vi "Init.vi"(11 "Game Play Type":refnum<vi>) -> (3 "cluster out":T1)   [LabVIEW 2019]
uses:
  Main VI references.ctl
  main queue data type.ctl
  top level commands.ctl
  error module commands.ctl
  Scene Commands.ctl
  Cube Data Ops.ctl
  Stop Timing Module commands.vi
  Play timing module commands.ctl
panel:
  in  "cluster":T1
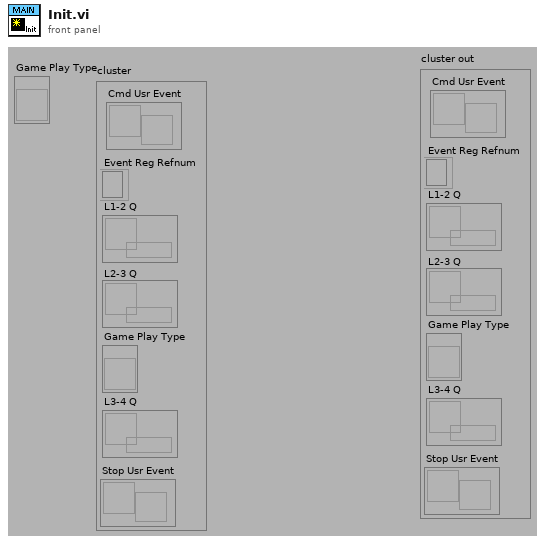
[diagram p1: front panel]
types:
  T1 = typedef "Main VI references.ctl" = cluster{"Cmd Usr Event":refnum<user-event>, "Event Reg Refnum":refnum<event-registration>, "L1-2 Q":refnum<queue>, "L2-3 Q":refnum<queue>, "Game Play Type":refnum<vi>, "L3-4 Q":refnum<queue>, "Stop Usr Event":refnum<user-event>}
  T2 = typedef "error module commands.ctl" = enum16{"Cleanup References", "Set References", "Report Errors", "Process Errors"}
  T3 = typedef "Scene Commands.ctl" = enum16{"Init", "Set Rubix Text Array", "Get Rubix Ref Array", "Generate Rubix Array", "Get Rubix Array", "Show Render Window", "Go To Face", "Rotate", "Update Scene", "Clear Rubix"}
  T4 = typedef "Play timing module commands.ctl" = enum16{"Clean up", "Initialize", "Run"}
  T5 = typedef "Cube Data Ops.ctl" = enum16{"Initialize", "Set Rubix Ref Array", "Set Rubix Text Array", "Set Current Face", "Get Rubix Text Array", "Generate Rubix Array", "Get Rubix array", "Get Facets to move", "Randomize", "Top row left", "Top row right", "Middle row left", "Middle row right", "Bottom row left", "Bottom row right", "Left column up", "Left column down", "Middle column up", "Middle column down", "Right column up", "Right column down", "Face ccw", "Face cw"}
  T6 = typedef "Stop Timing Module commands.vi" = enum16{"Set Name", "Stop loops"}
  T7 = typedef "main queue data type.ctl" = cluster{"Command":T8, "Data":variant}
  T8 = typedef "top level commands.ctl" = enum16{"Idle", "Set Cube Orientation", "Get Cube Orientation", "Go to Face", "Solve", "Test", "Randomize", "Game Play Type", "Stop", "rotate Cube"}
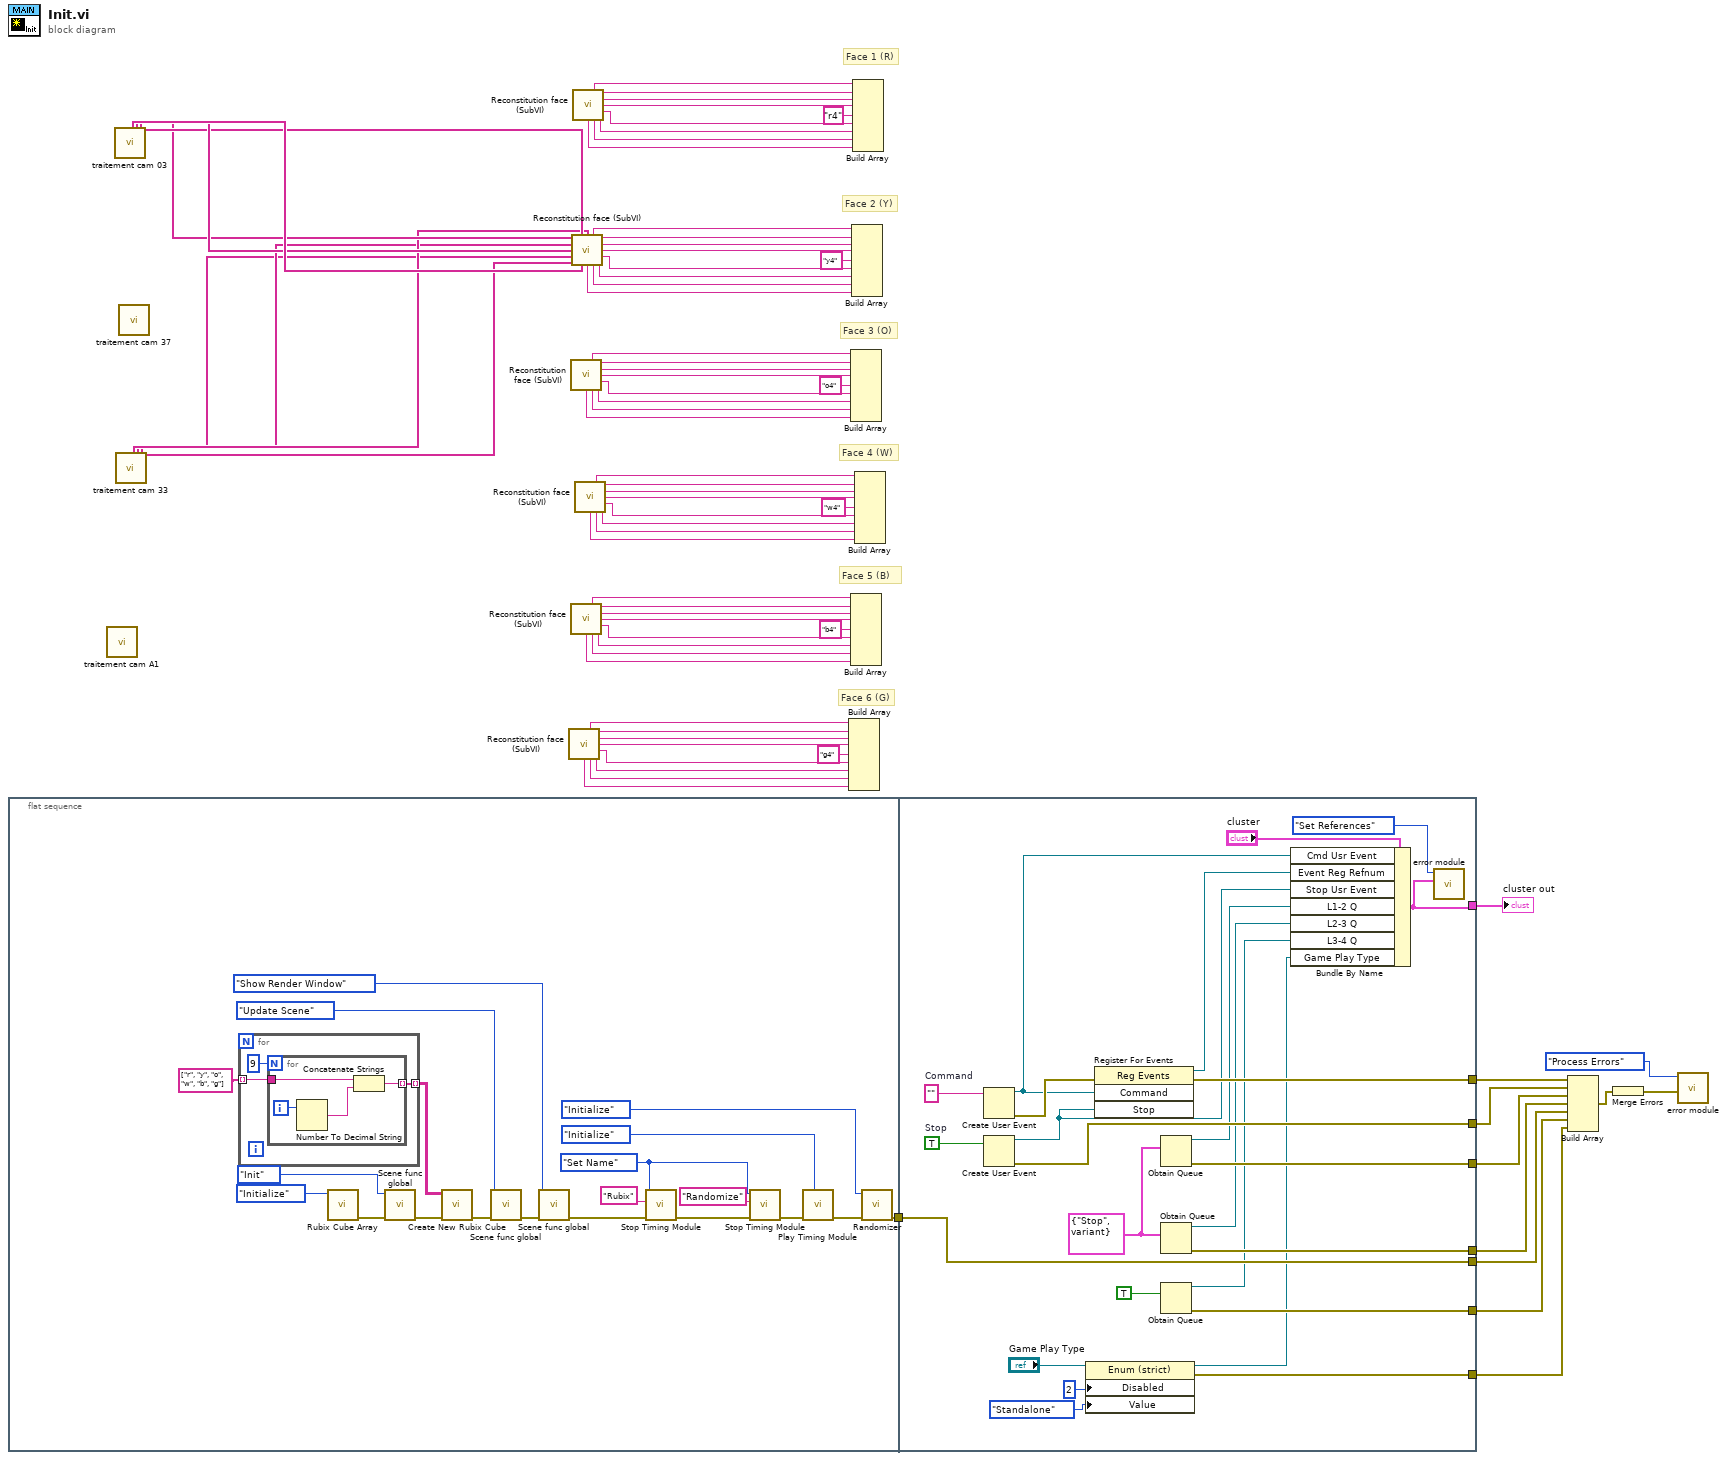
[diagram p0: block diagram]
diagram:
  # "Face 6 (G)"
  # "Face 5 (B)"
  # "Face 4 (W)"
  # "Face 3 (O)"
  # "Face 2 (Y)"
  # "Face 1 (R)"
  n1 = flat-sequence {
    tunnel: [w77] -> w68
    tunnel: [w118] -> w74
    tunnel: [w117] -> w72
    tunnel: [w116] -> w71
    tunnel: [w115] -> w70
    tunnel: [w103] -> w63
    tunnel: [w114] -> w73
    tunnel: [w113] -> w67
    tunnel: w68 -> [w113]
    tunnel: [w104] -> w66
    frame #0 {
      w87 = Stop_Timing_Module_commands.vi."Set Name" ("command")
      n2 = for {
        tunnel: string[] ["r", "y", "o", "w", "b", "g"] -> [w97] mode=indexing
        tunnel: [w95] -> w75 mode=indexing
        n3 = for {
          N: 9 -> [_]
          tunnel: w97 -> [w100]
          tunnel: [w98] -> w95 mode=indexing
          i -> [w101]
          n4 = Number To Decimal String(number=w101) -> (decimal integer string=w99:string)  [unwired: 1 in]
          n5 = Concatenate Strings(w100, w99) -> (w98:string)
        }
      }
      n6 = call "Rubix Cube Array.vi"("Command"=Cube_Data_Ops."Initialize") -> ("error out(no error)"=w92:errorcluster)  [unwired: 6 in, 4 out]
      n7 = call "Scene func global.vi"("error in (no error)"=w92, "Commands"=Scene_Commands."Init") -> ("error out"=w83:errorcluster)  [unwired: 8 in, 1 out]
      n8 = call "Create New Rubix Cube.vi"("error out"=w83, "Rubix Array pattern"=w75) -> ("error out(no error)"=w81:errorcluster)  [unwired: 9 in]
      n9 = call "Scene func global.vi"("error in (no error)"=w81, "Commands"=Scene_Commands."Update Scene") -> ("error out"=w79:errorcluster)  [unwired: 8 in, 1 out]
      n10 = call "Scene func global.vi"("error in (no error)"=w79, "Commands"=Scene_Commands."Show Render Window") -> ("error out"=w78:errorcluster)  [unwired: 8 in, 1 out]
      n11 = call "Stop Timing Module.vi"("error in (no error)"=w78, "Structure Names"="Rubix", "command"=w87) -> ("error out"=w89:errorcluster)  [unwired: 8 in]
      n12 = call "Stop Timing Module.vi"("error in (no error)"=w89, "Structure Names"="Randomize", "command"=w87) -> ("error out"=w88:errorcluster)  [unwired: 8 in]
      n13 = call "Play Timing Module.vi"("Commands"=Play_timing_module_commands."Initialize", "error in"=w88) -> ("error out"=w84:errorcluster)  [unwired: 9 in]
      n14 = call "Randomizer.vi"("error in"=w84, "Commands"=Play_timing_module_commands."Initialize") -> ("error out"=w77:errorcluster)  [unwired: 9 in]
    }
    frame #1 {
      w126 = ""  # Command
      w125 = TRUE  # Stop
      w123 = T7 {"Command"=enum."Stop", "Data"=variant} ("Cluster")
      n15 = Create User Event(user event datatype=w126) -> (user event=w110:refnum<user-event>, error out=w119:errorcluster)  [unwired: 1 in]
      n16 = Create User Event(user event datatype=w125) -> (user event=w106:refnum<user-event>, error out=w114:errorcluster)  [unwired: 1 in]
      n17 = property class="Enum (strict)"(reference="Game Play Type", "Disabled"=u8 2, "Value"=enum16{"Standalone", "UI Master", "UI Salve"}."Standalone") -> (reference out=w102:refnum<vi>, error out=w103:errorcluster)  [unwired: 1 in]
      n18 = register-events(error in=w119, w110, w106) -> (reference out=w111:refnum<event-registration>, error out=w118:errorcluster)  [unwired: 1 in]
      n19 = Obtain Queue(element data type=w123) -> (queue out=w109:refnum<queue>, error out=w117:errorcluster)  [unwired: 4 in, 1 out]
      n20 = Obtain Queue(element data type=w123) -> (queue out=w108:refnum<queue>, error out=w116:errorcluster)  [unwired: 4 in, 1 out]
      n21 = Obtain Queue(element data type=TRUE) -> (queue out=w107:refnum<queue>, error out=w115:errorcluster)  [unwired: 4 in, 1 out]
      n22 = Bundle By Name(cluster="cluster", "Cmd Usr Event"=w110, "Event Reg Refnum"=w111, "Stop Usr Event"=w106, "L1-2 Q"=w109, "L2-3 Q"=w108, "L3-4 Q"=w107, "Game Play Type"=w102) -> (w104:T1)
      n23 = call "error module.vi"("cluster 2"=w104, "Enum"=error_module_commands."Set References") -> ()  [unwired: 9 in, 1 out]
    }
  }
  n24 = call "traitement cam A1.vi"() -> ()  [unwired: 15 in, 13 out]
  n25 = call "traitement cam 03.vi"() -> ("Couleur carré 4 (2,9)"=w8:string[], "Couleur carré 3 (2,6)"=w7:string[], "Couleur carré 2 (2,3)"=w5:string[], "Couleur carré 1 (2,2)"=w6:string[])  [unwired: 15 in, 9 out]
  n26 = call "traitement cam 33.vi"() -> ("Couleur carré 4 (2,1)"=w4:string[], "Couleur carré 3 (2,4)"=w3:string[], "Couleur carré 2 (2,7)"=w2:string[], "Couleur carré 1 (2,8)"=w1:string[])  [unwired: 15 in, 9 out]
  n27 = call "traitement cam 37.vi"() -> ()  [unwired: 15 in, 13 out]
  n28 = call "Reconstitution face (SubVI).vi"() -> ("Couleur 0"=w9:string, "Couleur 1"=w10:string, "Couleur  2"=w11:string, "Couleur 3"=w12:string, "Couleur 5"=w13:string, "Couleur 8"=w15:string, "Couleur 7"=w16:string, "Couleur 6"=w14:string)  [unwired: 8 in]
  n29 = call "Reconstitution face (SubVI).vi"() -> ("Couleur 0"=w44:string, "Couleur 1"=w43:string, "Couleur  2"=w42:string, "Couleur 3"=w41:string, "Couleur 5"=w40:string, "Couleur 8"=w38:string, "Couleur 7"=w37:string, "Couleur 6"=w39:string)  [unwired: 8 in]
  n30 = call "Reconstitution face (SubVI).vi"() -> ("Couleur 0"=w26:string, "Couleur 1"=w25:string, "Couleur  2"=w24:string, "Couleur 3"=w23:string, "Couleur 5"=w22:string, "Couleur 8"=w20:string, "Couleur 7"=w19:string, "Couleur 6"=w21:string)  [unwired: 8 in]
  n31 = call "Reconstitution face (SubVI).vi"("Couleur carrée  2"=w5, "Couleur carrée  1"=w6, "Couleur carrée 0"=w4, "Couleur carrée  3"=w3, "Couleur carrée  5"=w7, "Couleur carrée  6"=w2, "Couleur carrée  7"=w1, "Couleur carrée  8"=w8) -> ("Couleur 0"=w45:string, "Couleur 1"=w46:string, "Couleur  2"=w47:string, "Couleur 3"=w48:string, "Couleur 5"=w49:string, "Couleur 8"=w51:string, "Couleur 7"=w52:string, "Couleur 6"=w50:string)
  n32 = call "Reconstitution face (SubVI).vi"() -> ("Couleur 0"=w62:string, "Couleur 1"=w61:string, "Couleur  2"=w60:string, "Couleur 3"=w59:string, "Couleur 5"=w58:string, "Couleur 8"=w56:string, "Couleur 7"=w55:string, "Couleur 6"=w57:string)  [unwired: 8 in]
  n33 = call "Reconstitution face (SubVI).vi"() -> ("Couleur 0"=w27:string, "Couleur 1"=w28:string, "Couleur  2"=w29:string, "Couleur 3"=w30:string, "Couleur 5"=w31:string, "Couleur 8"=w33:string, "Couleur 7"=w34:string, "Couleur 6"=w32:string)  [unwired: 8 in]
  n34 = Build Array(w9, w10, w11, w12, "g4" ("element"), w13, w14, w16, w15) -> ()  [unwired: 1 out]
  n35 = Build Array(w44, w43, w42, w41, "o4" ("element"), w40, w39, w37, w38) -> ()  [unwired: 1 out]
  n36 = Build Array(w26, w25, w24, w23, "b4" ("element"), w22, w21, w19, w20) -> ()  [unwired: 1 out]
  n37 = Build Array(w45, w46, w47, w48, "y4" ("element"), w49, w50, w52, w51) -> ()  [unwired: 1 out]
  n38 = Build Array(w62, w61, w60, w59, "r4" ("element"), w58, w57, w55, w56) -> ()  [unwired: 1 out]
  n39 = Build Array(w27, w28, w29, w30, "w4" ("element"), w31, w32, w34, w33) -> ()  [unwired: 1 out]
  n40 = Build Array(w74, w73, w72, w71, w67, w70, w63) -> (w69:errorcluster[])
  n41 = Merge Errors(w69) -> (w65:errorcluster)
  n42 = call "error module.vi"("error in (no error)"=w65, "Enum"=error_module_commands."Process Errors") -> ()  [unwired: 9 in, 1 out]
  "cluster out" <- w66
